vi "init.vi"(8 "error in (no error)":errorcluster, 11 "TTL input":T1) -> (0 "error out":errorcluster, 3 "TTL_input out":refnum<class "TTL_input.lvclass">)   [LabVIEW 2013, in "TTL_input.lvclass"]
uses:
  TTL_input.lvclass
  TTL_input_settings.ctl
  TTL_input.lvclass/TTL_input.ctl
  <vilib>/DAQmx/create/channels.llb/DAQmx Create Channel (DI-Digital Input).vi
  <vilib>/DAQmx/configure/timing.llb/DAQmx Timing (Sample Clock).vi
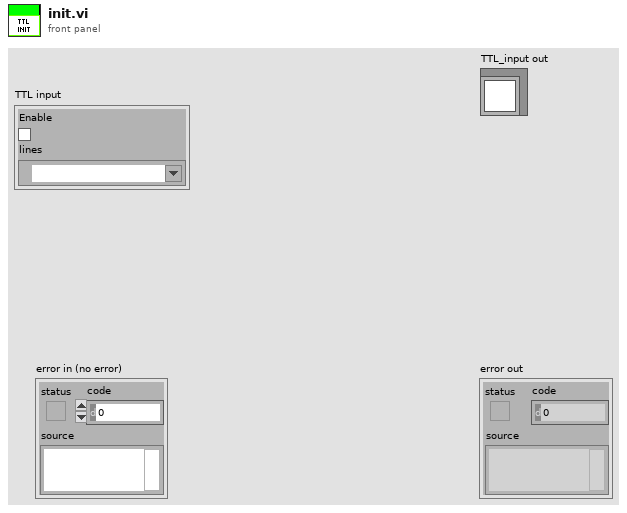
[diagram p1: front panel]
types:
  T1 = typedef "TTL_input.lvclass/TTL_input_settings.ctl" = cluster{"Enable":bool, "lines":tag}
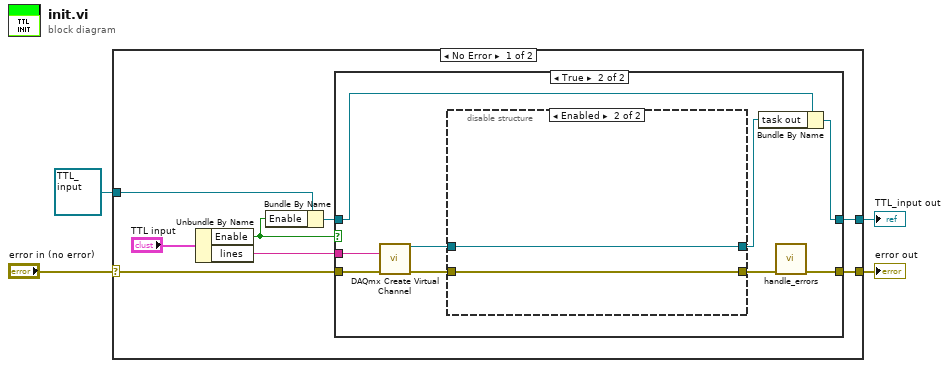
[diagram p0: block diagram]
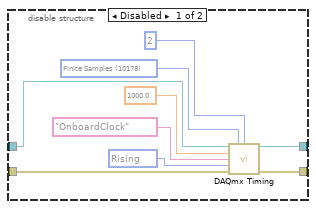
[diagram p3: hidden frame]
diagram:
  n1 = case shown="No Error" "error in (no error)" {
    selector: "error in (no error)" -> [w12 w36]
    tunnel: [w11 w36] -> w3
    tunnel: [w10 w35] -> w2
    tunnel: refnum<class "TTL_input.lvclass"> refnum ("TTL_input.lvclass") -> [w6 w35]
    frame No Error {
      n2 = Unbundle By Name("TTL input") -> ("Enable"=w7:bool, "lines"=w8:tag)
      n3 = Bundle By Name(cluster=w6, "Enable"=w7) -> (w5:refnum<class "TTL_input.lvclass">)
      n4 = case shown="True" w7 {
        tunnel: w12 -> [w13 w20]
        tunnel: [w13 w19] -> w11
        tunnel: w5 -> [w14 w18]
        tunnel: [w14 w17] -> w10
        tunnel: w8 -> [_ w15]
        frame False {
        }
        frame True {
          n5 = call-poly <vilib>:"DAQmx Create Virtual Channel.vi"("lines"=w15, "error in"=w20) -> ("task out"=w23:refnum<k21>, "error out"=w22:errorcluster)  [unwired: 12 in]
          n6 = disable-structure shown="Enabled" {
            disable-tunnel: w23 -> [w32 w34]
            disable-tunnel: w22 -> [w29 w33]
            disable-tunnel: [w28 w33] -> w21
            disable-tunnel: [w24 w34] -> w16
            frame Disabled {
              w25 = 10280 items=["Rising"=10280, "Falling"=10171] ("active edge")
              w30 = 10178 items=["Finite Samples"=10178, "Continuous Samples"=10123, "Hardware Timed Single Point"=12522] ("sample mode")
              n7 = call-poly <vilib>:"DAQmx Timing.vi"("task/channels in"=w32, "sample mode"=w30, "samples per channel"=2, "rate"=1000.0, "source"=tag "OnboardClock", "active edge"=w25, "error in"=w29) -> ("task out"=w24:refnum<k21>, "error out"=w28:errorcluster)  [unwired: 7 in]
            }
            frame Enabled {
            }
          }
          n8 = Bundle By Name(cluster=w18, "task out"=w16) -> (w17:refnum<class "TTL_input.lvclass">)
          n9 = call "handle_errors.vi"("error in (no error)"=w21) -> ("error out"=w19:errorcluster)  [unwired: 10 in]
        }
      }
    }
    frame Error {
    }
  }
  "error out" <- w3
  "TTL_input out" <- w2
